vi "Shut Down Device.vi"(8 "error in (no error)":errorcluster, 11 "ASI Stage in":refnum<class "ASI Stage.lvclass">) -> (0 "error out":errorcluster, 3 "ASI Stage out":refnum<class "ASI Stage.lvclass">)   [LabVIEW 2023, in "ASI Stage.lvlib" / "ASI Stage.lvclass"]
uses:
  ASI Stage.lvclass
  ASI Stage.lvclass/ASI Stage.ctl
  <instrlib>/ASI TG-1000/ASI TG-1000.lvlib
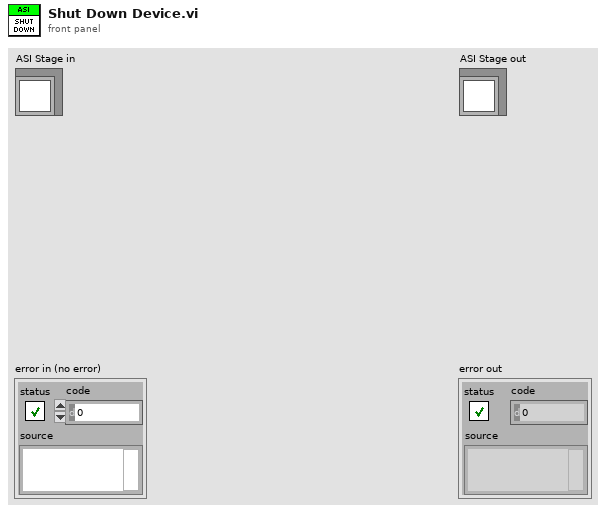
[diagram p1: front panel]
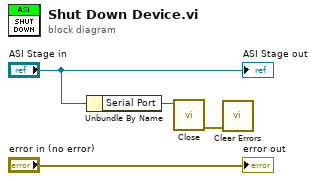
[diagram p0: block diagram]
diagram:
  n1 = Unbundle By Name("ASI Stage in") -> ("Serial Port"=w3:refnum<visa-resource-name>)
  n2 = call <instrlib>:"Close.vi"("VISA resource name"=w3) -> ("error out"=w1:errorcluster)  [unwired: 10 in]
  n3 = call <vilib>:"Clear Errors.vi"("error in (no error)"=w1) -> ()  [unwired: 5 in, 2 out]
  "error out" <- "error in (no error)"
  "ASI Stage out" <- "ASI Stage in"
